vi "main.vi"() -> ()   [LabVIEW 2020]
panel:
  out "Current S-HV":dbl
  out "Current Y-HV":dbl
  out "Current Z-HV":dbl
  out "Current X-HV":dbl
  in  "S(0.035~3)":dbl
  in  "Z(0.15~15)":dbl
  in  "Y(1.2~35)":dbl
  in  "X (1.2~35)":dbl
  in  "set Home velocity":bool
  in  "V INITISLIZE":bool
  out "Current S":dbl
  out "Current Z":dbl
  out "Current Y":dbl
  out "Current X":dbl
  in  "Set S(0.035~3)":dbl
  in  "Set Z(0.15~20)":dbl
  in  "Set Y(1.2~200)":dbl
  in  "Set X(1.2~200)":dbl
  in  "V set":bool
  in  "EXIT":bool
  out "error out":errorcluster
  in  "Axis-HOME":enum16{"X", "Y", "Z", "S"}(ring)
  out "Arrived -HOME":bool
  in  "Home":bool
  out "Arrived":bool
  out "Current Position(mm)":dbl
  in  "Occupied Length by Air(mm)":dbl=1.2 format="%#_13g"
  in  "Position(mm)":dbl
  in  "Axis":enum16{"X", "Y", "Z", "S"}(ring)
  in  "Go to the Position":bool
  in  "Connect":bool
  out "S Connecting":bool
  out "Z Connecting":bool
  out "Y Connecting":bool
  out "X  Connecting":bool
  in  "COM Port":refnum<visa-resource-name>
  # "Position :"
  # "Home/HOME velocity (mm/s) :"
  # "(set the Occupied length by Air if the target axis is syringe axis)"
  # "Velocity (mm/s) :"
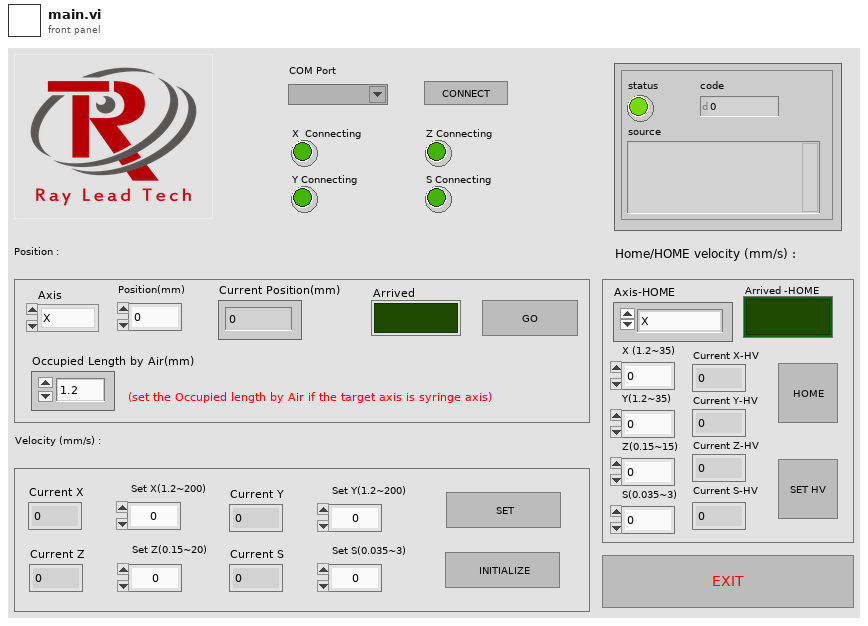
[diagram p1: front panel]
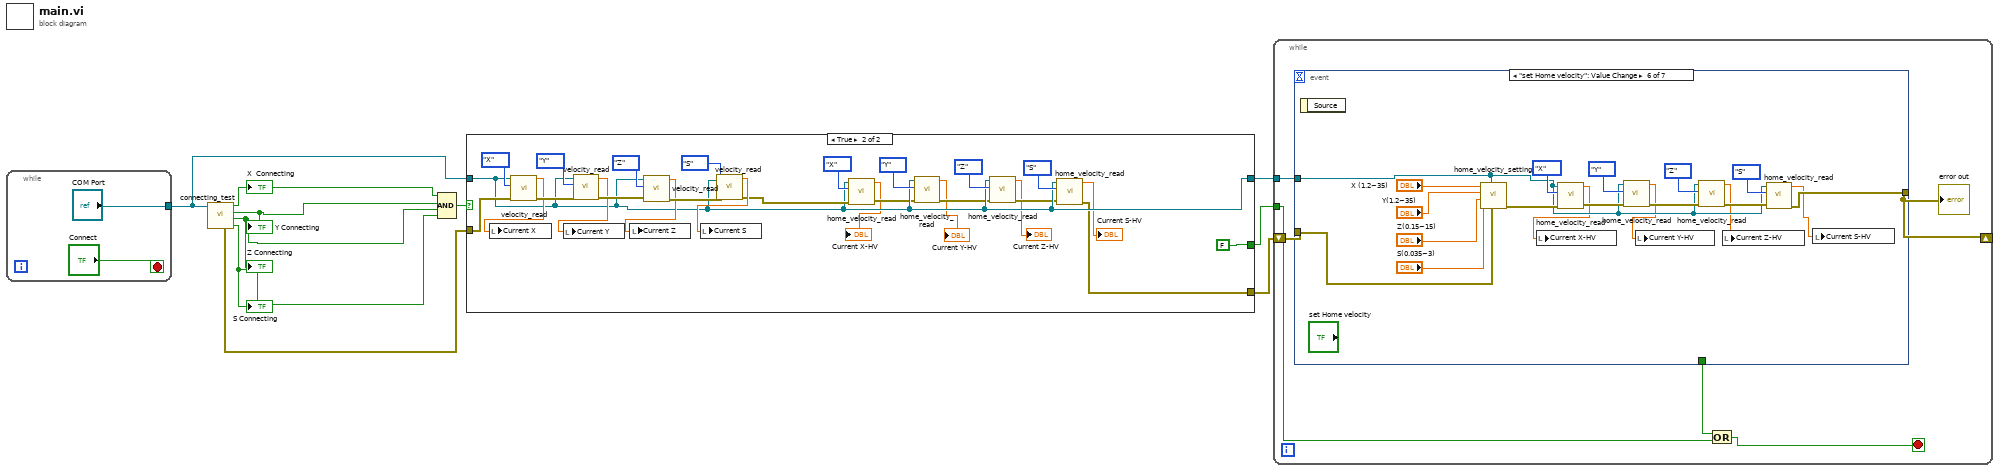
[diagram p0: block diagram]
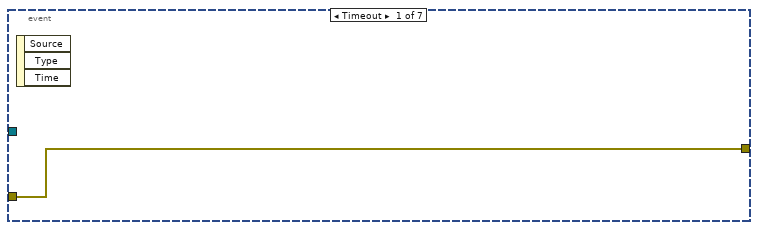
[diagram p2: hidden frame]
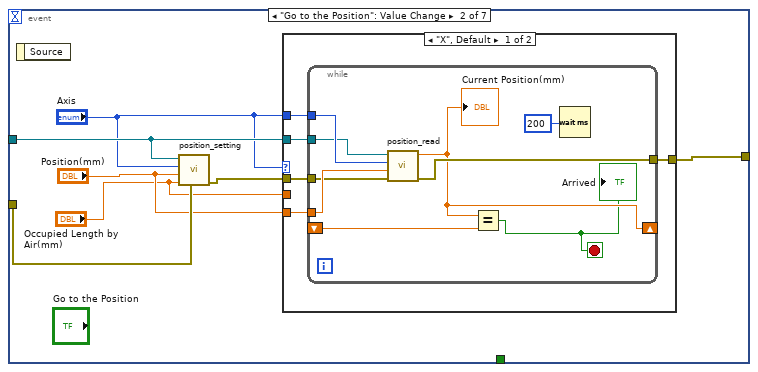
[diagram p3: hidden frame]
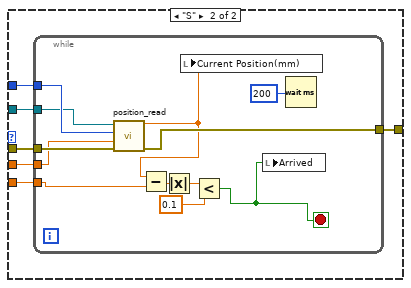
[diagram p4: hidden frame]
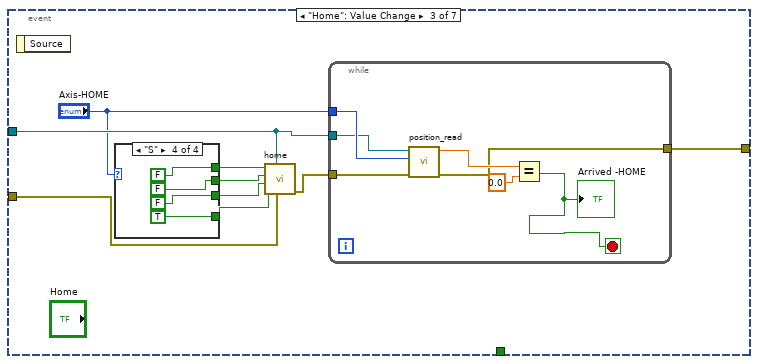
[diagram p5: hidden frame]
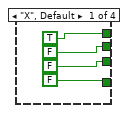
[diagram p6: hidden frame]
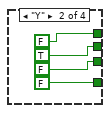
[diagram p7: hidden frame]
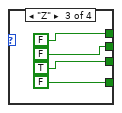
[diagram p8: hidden frame]
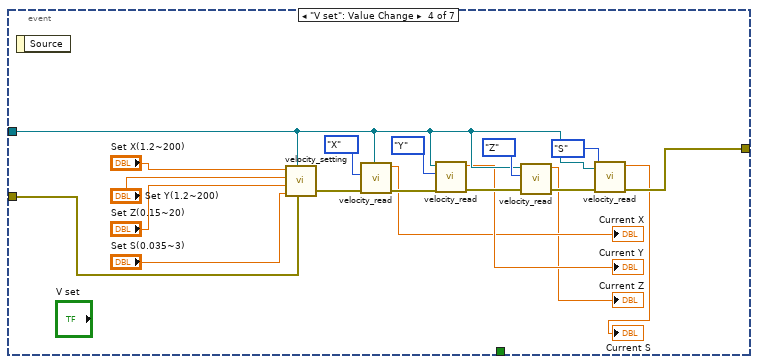
[diagram p9: hidden frame]
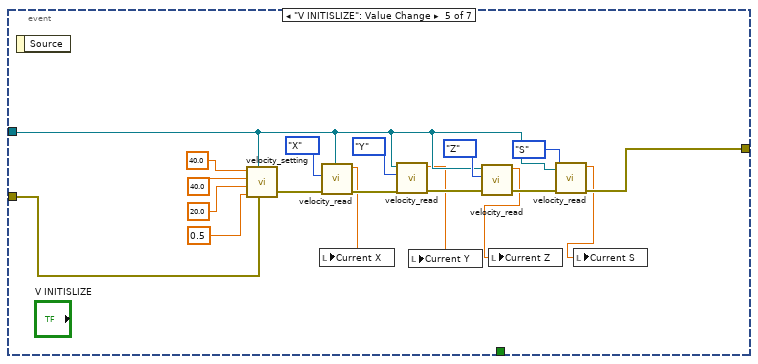
[diagram p10: hidden frame]
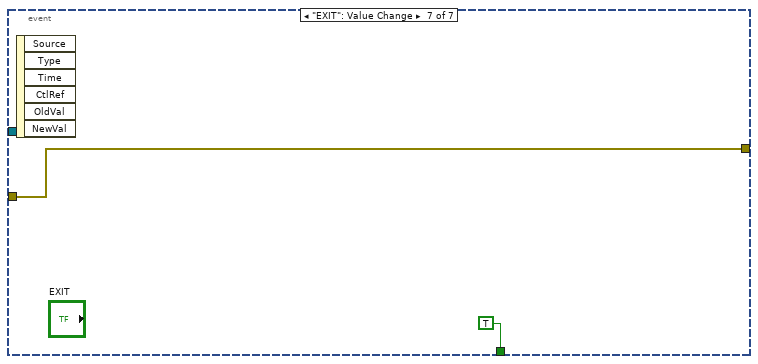
[diagram p11: hidden frame]
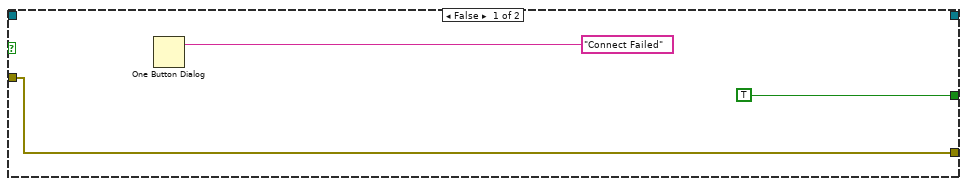
[diagram p12: hidden frame]
diagram:
  n1 = while {
    tunnel: ["COM Port"] -> w5
    stop <- "Connect" stop-if-true
  }
  n2 = call "connecting_test.vi"("VISA resource name"=w5) -> ("syringe axis connecting"=w7:bool, "Z axis connecting"=w8:bool, "Y axis connecting"=w9:bool, "X axis connecting"=w10:bool, "error out"=w2:errorcluster)  [unwired: 6 in]
  "X  Connecting" <- w10
  "Y Connecting" <- w9
  "Z Connecting" <- w8
  "S Connecting" <- w7
  n3 = Compound Arithmetic op=AND(w10, w9, w8, w7) -> (w6:bool)
  n4 = case shown="True" w6 {
    tunnel: w5 -> [_ w24]
    tunnel: [_ w24] -> w3
    tunnel: [TRUE FALSE] -> w4
    tunnel: w2 -> [w13 w40]
    tunnel: [w13 w20] -> w1
    frame False {
      n5 = One Button Dialog(message="Connect Failed") -> ()  [unwired: 1 in, 1 out]
    }
    frame True {
      n6 = call "velocity_read.vi"("error in (no error)"=w40, "Axis"=enum16{"X", "Y", "Z", "S"}."X", "COM Port"=w24) -> ("error out"=w39:errorcluster, "current velocity(mm/s)"=w33:dbl)  [unwired: 7 in]
      n7 = local write "Current X"(w33) -> ()
      n8 = call "velocity_read.vi"("error in (no error)"=w39, "Axis"=enum16{"X", "Y", "Z", "S"}."Y", "COM Port"=w24) -> ("error out"=w38:errorcluster, "current velocity(mm/s)"=w32:dbl)  [unwired: 7 in]
      n9 = local write "Current Y"(w32) -> ()
      n10 = call "velocity_read.vi"("error in (no error)"=w38, "Axis"=enum16{"X", "Y", "Z", "S"}."Z", "COM Port"=w24) -> ("error out"=w36:errorcluster, "current velocity(mm/s)"=w31:dbl)  [unwired: 7 in]
      n11 = local write "Current Z"(w31) -> ()
      n12 = call "velocity_read.vi"("error in (no error)"=w36, "Axis"=enum16{"X", "Y", "Z", "S"}."S", "COM Port"=w24) -> ("error out"=w28:errorcluster, "current velocity(mm/s)"=w30:dbl)  [unwired: 7 in]
      n13 = local write "Current S"(w30) -> ()
      n14 = call "home_velocity_read.vi"("error in (no error)"=w28, "Axis"=enum16{"X", "Y", "Z", "S"}."X", "COM Port"=w24) -> ("error out"=w23:errorcluster, "Current Home Velocity(mm/s)"=→"Current X-HV":dbl)  [unwired: 7 in]
      n15 = call "home_velocity_read.vi"("error in (no error)"=w23, "Axis"=enum16{"X", "Y", "Z", "S"}."Y", "COM Port"=w24) -> ("error out"=w22:errorcluster, "Current Home Velocity(mm/s)"=→"Current Y-HV":dbl)  [unwired: 7 in]
      n16 = call "home_velocity_read.vi"("error in (no error)"=w22, "Axis"=enum16{"X", "Y", "Z", "S"}."Z", "COM Port"=w24) -> ("error out"=w21:errorcluster, "Current Home Velocity(mm/s)"=→"Current Z-HV":dbl)  [unwired: 7 in]
      n17 = call "home_velocity_read.vi"("error in (no error)"=w21, "Axis"=enum16{"X", "Y", "Z", "S"}."S", "COM Port"=w24) -> ("error out"=w20:errorcluster, "Current Home Velocity(mm/s)"=→"Current S-HV":dbl)  [unwired: 7 in]
    }
  }
  n18 = while {
    tunnel: w4 -> [w48]
    tunnel: w3 -> [w47]
    shift-right: [w43] -> _
    shift-left: w1 -> [w44]
    stop <- w46 stop-if-true
    n19 = event shown="[5] \"set Home velocity\": Value Change" {
      selector: _ -> [_ _ _ _ _ _ _]
      dyn-events: _ -> [_ _ _ _ _ _ _]
      timeout: _ -> [_ _ _ _ _ _ _]
      tunnel: w47 -> [_ w56 w97 w128 w145 w164 _]
      tunnel: [_ _ _ _ _ _ TRUE] -> w45
      tunnel: [w49 w55 w91 w126 w144 w163 w178] -> w43
      tunnel: w44 -> [w49 w53 w89 w135 w146 w173 w178]
      event Timeout {
        n20 = event-data() -> ()  [unwired: 1 in, 3 out]
      }
      event "Go to the Position": Value Change {
        n21 = event-data() -> ()  [unwired: 1 in, 1 out]
        n22 = call "position_setting.vi"("error in (no error)"=w53, "Occupied length by Air(mm)"="Occupied Length by Air(mm)", "Distance(mm)"="Position(mm)", "Axis"="Axis", "Com Port"=w56) -> ("error out"=w54:errorcluster)  [unwired: 6 in]
        n23 = case shown="\"X\", Default" "Axis" {
          tunnel: "Axis" -> [w61 w76]
          tunnel: w56 -> [w60 w75]
          tunnel: "Position(mm)" -> [w59 w74]
          tunnel: [w58 w73] -> w55
          tunnel: w54 -> [w57 w72]
          tunnel: "Occupied Length by Air(mm)" -> [_ w71]
          frame "X", Default {
            n24 = while {
              tunnel: w60 -> [w69]
              tunnel: w61 -> [w70]
              tunnel: w59 -> [w68]
              tunnel: [w67] -> w58
              tunnel: w57 -> [w66]
              shift-right: [w64] -> _
              shift-left: _ -> [w65]
              stop <- w62 stop-if-true
              n25 = call "position_read.vi"("error in (no error)"=w66, "Occupied Length by Air(mm)"=w68, "Axis"=w70, "COM Port"=w69) -> ("error out"=w67:errorcluster, "current position(mm)"=w64:dbl)  [unwired: 6 in]
              "Current Position(mm)" <- w64
              n26 = Equal?(x=w64, y=w65) -> (x = y?=w62:bool)
              "Arrived" <- w62
              n27 = Wait (ms)(milliseconds to wait=u32 200) -> ()  [unwired: 1 out]
            }
          }
          frame "S" {
            n28 = while {
              tunnel: w75 -> [w87]
              tunnel: w76 -> [w88]
              tunnel: w74 -> [w82]
              tunnel: [w86] -> w73
              tunnel: w72 -> [w85]
              tunnel: w71 -> [w77]
              stop <- w78 stop-if-true
              n29 = call "position_read.vi"("error in (no error)"=w85, "Occupied Length by Air(mm)"=w77, "Axis"=w88, "COM Port"=w87) -> ("error out"=w86:errorcluster, "current position(mm)"=w83:dbl)  [unwired: 6 in]
              n30 = Subtract(x=w83, y=w82) -> (x-y=w81:dbl)
              n31 = Absolute Value(x=w81) -> (abs(x)=w80:dbl)
              n32 = local write "Current Position(mm)"(w83) -> ()
              n33 = Less?(x=w80, y=0.1) -> (x < y?=w78:bool)
              n34 = local write "Arrived"(w78) -> ()
              n35 = Wait (ms)(milliseconds to wait=u32 200) -> ()  [unwired: 1 out]
            }
          }
        }
      }
      event "Home": Value Change {
        n36 = event-data() -> ()  [unwired: 1 in, 1 out]
        n37 = case shown="\"S\"" "Axis-HOME" {
          tunnel: [TRUE FALSE FALSE FALSE] -> w95
          tunnel: [FALSE TRUE FALSE FALSE] -> w94
          tunnel: [FALSE FALSE TRUE FALSE] -> w93
          tunnel: [FALSE FALSE FALSE TRUE] -> w92
          frame "X", Default {
          }
          frame "Y" {
          }
          frame "Z" {
          }
          frame "S" {
          }
        }
        n38 = call "home.vi"("error in (no error)"=w89, "COM Port"=w97, "Syringe axis stop"=w92, "Z axis stop"=w93, "Y axis stop"=w94, "X axis stop"=w95) -> ("error out"=w90:errorcluster)  [unwired: 5 in]
        n39 = while {
          tunnel: w97 -> [w119]
          tunnel: "Axis-HOME" -> [w120]
          tunnel: [w115] -> w91
          tunnel: w90 -> [w114]
          stop <- w116 stop-if-true
          n40 = call "position_read.vi"("error in (no error)"=w114, "Axis"=w120, "COM Port"=w119) -> ("error out"=w115:errorcluster, "current position(mm)"=w117:dbl)  [unwired: 7 in]
          n41 = Equal?(x=w117, y=0.0) -> (x = y?=w116:bool)
          "Arrived -HOME" <- w116
        }
      }
      event "V set": Value Change {
        n42 = event-data() -> ()  [unwired: 1 in, 1 out]
        n43 = call "velocity_setting.vi"("error in (no error)"=w135, "COM Port"=w128, "Syringe velocity (mm/s)"="Set S(0.035~3)", "Z velocity (mm/s)"="Set Z(0.15~20)", "Y velocity (mm/s)"="Set Y(1.2~200)", "X velocity (mm/s)"="Set X(1.2~200)") -> ("error out"=w125:errorcluster)  [unwired: 5 in]
        n44 = call "velocity_read.vi"("error in (no error)"=w125, "Axis"=enum16{"X", "Y", "Z", "S"}."X", "COM Port"=w128) -> ("error out"=w133:errorcluster, "current velocity(mm/s)"=→"Current X":dbl)  [unwired: 7 in]
        n45 = call "velocity_read.vi"("error in (no error)"=w133, "Axis"=enum16{"X", "Y", "Z", "S"}."Y", "COM Port"=w128) -> ("error out"=w132:errorcluster, "current velocity(mm/s)"=→"Current Y":dbl)  [unwired: 7 in]
        n46 = call "velocity_read.vi"("error in (no error)"=w132, "Axis"=enum16{"X", "Y", "Z", "S"}."Z", "COM Port"=w128) -> ("error out"=w127:errorcluster, "current velocity(mm/s)"=→"Current Z":dbl)  [unwired: 7 in]
        n47 = call "velocity_read.vi"("error in (no error)"=w127, "Axis"=enum16{"X", "Y", "Z", "S"}."S", "COM Port"=w128) -> ("error out"=w126:errorcluster, "current velocity(mm/s)"=→"Current S":dbl)  [unwired: 7 in]
      }
      event "V INITISLIZE": Value Change {
        n48 = event-data() -> ()  [unwired: 1 in, 1 out]
        n49 = call "velocity_setting.vi"("error in (no error)"=w146, "COM Port"=w145, "Syringe velocity (mm/s)"=0.5 ("Set S  2"), "Z velocity (mm/s)"=20.0 ("Set Z  2"), "Y velocity (mm/s)"=40.0 ("Set Y  2"), "X velocity (mm/s)"=40.0 ("Set X   2")) -> ("error out"=w147:errorcluster)  [unwired: 5 in]
        n50 = call "velocity_read.vi"("error in (no error)"=w147, "Axis"=enum16{"X", "Y", "Z", "S"}."X", "COM Port"=w145) -> ("error out"=w153:errorcluster, "current velocity(mm/s)"=w143:dbl)  [unwired: 7 in]
        n51 = local write "Current X"(w143) -> ()
        n52 = call "velocity_read.vi"("error in (no error)"=w153, "Axis"=enum16{"X", "Y", "Z", "S"}."Y", "COM Port"=w145) -> ("error out"=w152:errorcluster, "current velocity(mm/s)"=w142:dbl)  [unwired: 7 in]
        n53 = local write "Current Y"(w142) -> ()
        n54 = call "velocity_read.vi"("error in (no error)"=w152, "Axis"=enum16{"X", "Y", "Z", "S"}."Z", "COM Port"=w145) -> ("error out"=w148:errorcluster, "current velocity(mm/s)"=w141:dbl)  [unwired: 7 in]
        n55 = local write "Current Z"(w141) -> ()
        n56 = call "velocity_read.vi"("error in (no error)"=w148, "Axis"=enum16{"X", "Y", "Z", "S"}."S", "COM Port"=w145) -> ("error out"=w144:errorcluster, "current velocity(mm/s)"=w140:dbl)  [unwired: 7 in]
        n57 = local write "Current S"(w140) -> ()
      }
      event "set Home velocity": Value Change {
        n58 = event-data() -> ()  [unwired: 1 in, 1 out]
        n59 = call "home_velocity_setting.vi"("error in (no error)"=w173, "COM Port"=w164, "Syringe home velocity (mm/s)"="S(0.035~3)", "Z home velocity (mm/s)"="Z(0.15~15)", "Y home velocity (mm/s)"="Y(1.2~35)", "X home velocity (mm/s)"="X (1.2~35)") -> ("error out"=w165:errorcluster)  [unwired: 5 in]
        n60 = call "home_velocity_read.vi"("error in (no error)"=w165, "Axis"=enum16{"X", "Y", "Z", "S"}."X", "COM Port"=w164) -> ("error out"=w168:errorcluster, "Current Home Velocity(mm/s)"=w162:dbl)  [unwired: 7 in]
        n61 = local write "Current X-HV"(w162) -> ()
        n62 = call "home_velocity_read.vi"("error in (no error)"=w168, "Axis"=enum16{"X", "Y", "Z", "S"}."Y", "COM Port"=w164) -> ("error out"=w167:errorcluster, "Current Home Velocity(mm/s)"=w161:dbl)  [unwired: 7 in]
        n63 = local write "Current Y-HV"(w161) -> ()
        n64 = call "home_velocity_read.vi"("error in (no error)"=w167, "Axis"=enum16{"X", "Y", "Z", "S"}."Z", "COM Port"=w164) -> ("error out"=w166:errorcluster, "Current Home Velocity(mm/s)"=w160:dbl)  [unwired: 7 in]
        n65 = local write "Current Z-HV"(w160) -> ()
        n66 = call "home_velocity_read.vi"("error in (no error)"=w166, "Axis"=enum16{"X", "Y", "Z", "S"}."S", "COM Port"=w164) -> ("error out"=w163:errorcluster, "Current Home Velocity(mm/s)"=w159:dbl)  [unwired: 7 in]
        n67 = local write "Current S-HV"(w159) -> ()
      }
      event "EXIT": Value Change {
        n68 = event-data() -> ()  [unwired: 1 in, 6 out]
      }
    }
    "error out" <- w43
    n69 = Compound Arithmetic op=OR(w45, w48) -> (w46:bool)
  }
